vi "customised_subPlayWaveform.vi"(0 "Device":u32, 1 "Resolution (bits)":i32=16, 2 "Sample rate (Hz)":dbl=22050.0, 3 "Use rate":bool, 4 "Path":path, 5 "error in (no error)":errorcluster, 7 "Data":dynamicdata(waveform), 9 "Timeout (sec)":dbl=-1.0) -> (19 "error out":errorcluster)   [LabVIEW 2010]
uses:
  <vilib>/sound2/lvsound2.llb/Sound Output Write Simple (DBL2).vi
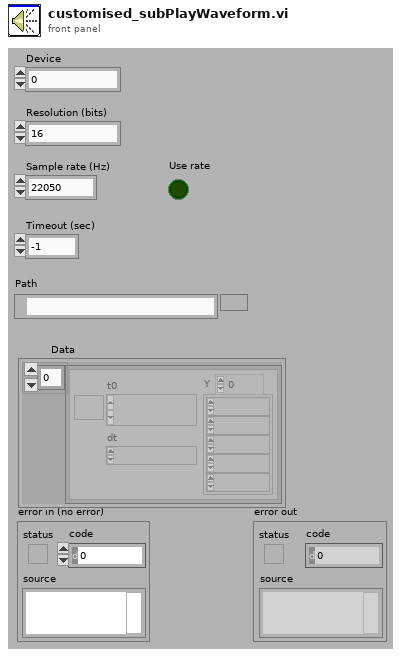
[diagram p1: front panel]
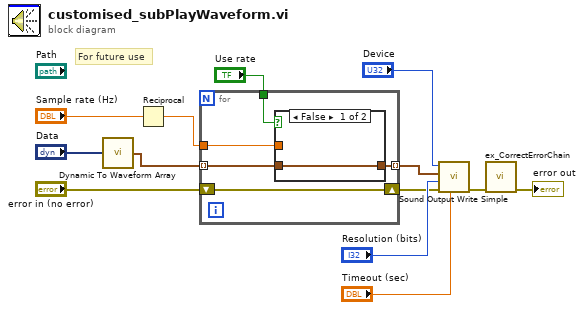
[diagram p0: block diagram]
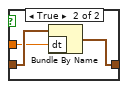
[diagram p2: hidden frame]
diagram:
  # "For future use"
  n1 = call <vilib>:"Dynamic To Waveform Array.vi"("Input"="Data") -> ("Output"=w5:waveform(dbl)[])  [unwired: 4 in]
  n2 = Reciprocal(x="Sample rate (Hz)") -> (1/x=w4:dbl)
  n3 = for {
    tunnel: w5 -> [w15] mode=indexing
    tunnel: [w17] -> w12 mode=indexing
    shift-right: [w14] -> w10
    shift-left: "error in (no error)" -> [w14]
    tunnel: "Use rate" -> [w18]
    tunnel: w4 -> [w16]
    n4 = case shown="False" w18 {
      tunnel: w15 -> [w19 w22]
      tunnel: [w19 w21] -> w17
      tunnel: w16 -> [_ w20]
      frame False {
      }
      frame True {
        n5 = Bundle By Name(cluster=w22, "dt"=w20) -> (w21:waveform(dbl))
      }
    }
  }
  n6 = call-poly <vilib>:"Sound Output Write Simple.vi"("timeout (sec)"="Timeout (sec)", "error in (no error)"=w10, "bits per sample"="Resolution (bits)", "data"=w12, "device ID"="Device") -> ("error out"=w2:errorcluster)  [unwired: 6 in]
  n7 = call <vilib>:"ex_CorrectErrorChain.vi"("error in (no error)"=w2) -> ("error out"=→"error out":errorcluster)  [unwired: 10 in]
